vi "Init Input.vi"(8 "error in (no error)":errorcluster, 10 "Descriptor":string, 11 "input in":refnum<class "Input.lvclass">) -> (0 "error out":errorcluster, 3 "input out":refnum<class "Input.lvclass">)   [LabVIEW 2015, in "Input.lvclass"]
uses:
  Input.lvclass
  Input.lvclass/Input.ctl
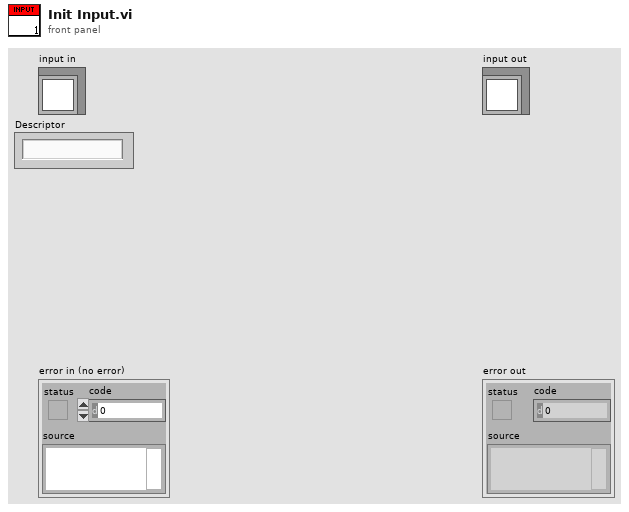
[diagram p1: front panel]
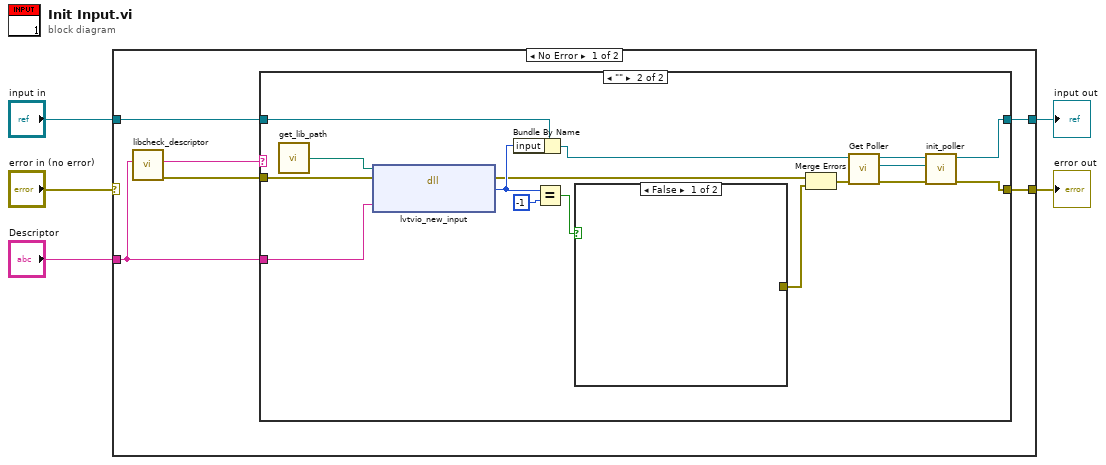
[diagram p0: block diagram]
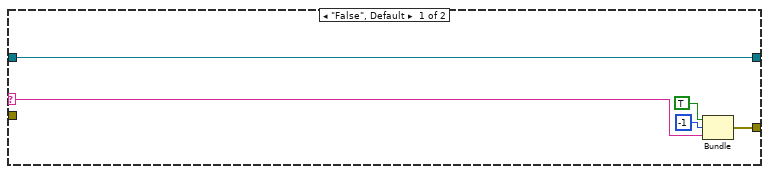
[diagram p2: hidden frame]
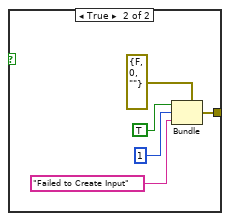
[diagram p3: hidden frame]
diagram:
  n1 = case shown="No Error" "error in (no error)" {
    selector: "error in (no error)" -> [_ w39]
    tunnel: [w11 w39] -> w4
    tunnel: [w10 w38] -> w2
    tunnel: "input in" -> [w9 w38]
    tunnel: "Descriptor" -> [w7 _]
    frame No Error {
      n2 = call "libcheck_descriptor.vi"("Descriptor"=w7) -> ("error out"=w8:errorcluster, "result"=w6:string)  [unwired: 9 in]
      n3 = case shown="\"\"" w6 {
        selector: w6 -> [w14 _]
        tunnel: [w13 w22] -> w11
        tunnel: [w12 w21] -> w10
        tunnel: w9 -> [w12 w18]
        tunnel: w8 -> [_ w20]
        tunnel: w7 -> [_ w19]
        frame "False", Default {
          n4 = Bundle("status"=TRUE, "code"=-1, w14) -> (w13:cluster{"status":bool, "code":i32, string})  [unwired: 1 in]
        }
        frame "" {
          n5 = call "get_lib_path.vi"() -> ("Path"=w28:path)
          n6 = dll-call lib="F:/lv-thingiverseio/lib/win_x86/liblvtvio.dll" fn="lvtvio_new_input"(path in=w28, error in=w20, "descriptor"=w19) -> (error out=w26:errorcluster, "return type"=w27:i32)  [unwired: 2 in, 1 out]
          n7 = Bundle By Name(cluster=w18, "input"=w27) -> (w17:refnum<class "Input.lvclass">)
          n8 = Equal?(x=w27, y=-1) -> (x = y?=w24:bool)
          n9 = case shown="False" w24 {
            tunnel: [_ w33] -> w25
            frame False {
            }
            frame True {
              n10 = Bundle(cluster=errorcluster {"status"=FALSE, "code"=0, "source"=""} ("error in (no error)"), "status"=TRUE, "code"=1, "source"="Failed to Create Input") -> (w33:errorcluster)
            }
          }
          n11 = Merge Errors(w26, w25) -> (w30:errorcluster)
          n12 = call-dynamic "Get Poller.vi"("error in (no error)"=w30, "input in"=w17) -> ("error out"=w31:errorcluster, "input_poller.lvclass"=w32:refnum<class "input_poller.lvclass">, "input out"=w29:refnum<class "Input.lvclass">)  [unwired: 7 in]
          n13 = call "init_poller.vi"("error in (no error)"=w31, "input_poller in"=w32, "input in"=w29) -> ("error out"=w22:errorcluster, "input out"=w21:refnum<class "Input.lvclass">)  [unwired: 7 in]
        }
      }
    }
    frame Error {
    }
  }
  "error out" <- w4
  "input out" <- w2
